vi "RSZVB Get Stop Frequency.vi"(8 "error in (no error)":errorcluster {"code" format="%.0x"}, 10 "Channel (1)":i32=1, 11 "VISA session":refnum<visa-resource-name>) -> (0 "error out":errorcluster {"code" format="%.0x"}, 2 "Stop Frequency":dbl format="%^.3e", 3 "dup VISA session":refnum<visa-resource-name>)   [LabVIEW 2011]
doc: "This VI queries the stop frequency for a frequency sweep which is equal to the right edge of a Cartesian diagram.\n\nRemote-control command(s):\n[SENSe<Ch>:]FREQuency:STOP?"
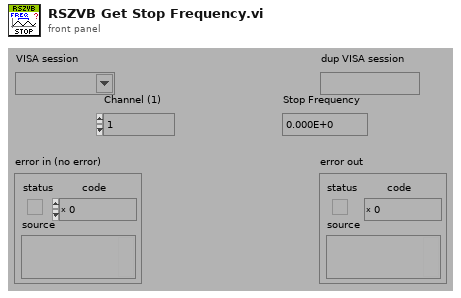
[diagram p1: front panel]
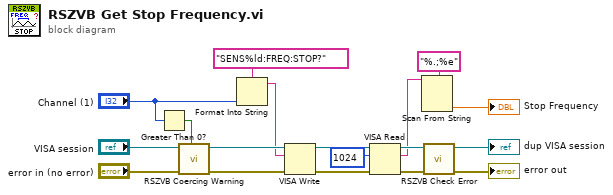
[diagram p0: block diagram]
diagram:
  n1 = Greater Than 0?(x="Channel (1)") -> (x > 0?=w14:bool)
  n2 = call "RSZVB Coercing Warning.vi"("In Range?"=w14, "error in (no error)"="error in (no error)", "VISA session"="VISA session") -> ("error out"=w16:errorcluster, "dup VISA session"=w17:refnum<visa-resource-name>)  [unwired: 7 in]
  n3 = Format Into String(format string="SENS%ld:FREQ:STOP?", "Channel (1)") -> (resulting string=w15:string)  [unwired: 2 in, 1 out]
  n4 = VISA Write(VISA resource name=w17, write buffer=w15, error in (no error)=w16) -> (VISA resource name out=w7:refnum<visa-resource-name>, error out=w8:errorcluster)  [unwired: 1 out]
  n5 = VISA Read(VISA resource name=w7, byte count=u32 1024 ("byte count (0)"), error in (no error)=w8) -> (VISA resource name out=w12:refnum<visa-resource-name>, read buffer=w9:string, error out=w11:errorcluster)  [unwired: 1 out]
  n6 = Scan From String(format string="%.;%e", input string=w9) -> (output 1=→"Stop Frequency":dbl)  [unwired: 3 in, 3 out]
  n7 = call "RSZVB Check Error.vi"("error in (no error)"=w11, "VISA session"=w12) -> ("error out"=→"error out":errorcluster, "dup VISA session"=→"dup VISA session":refnum<visa-resource-name>)  [unwired: 8 in]
